vi "MaxX_FITSstacks.vi"() -> ()   [LabVIEW 2011]
panel:
  in  "Skip left":dbl=0.1 min=0.0 max=0.999
  out "error out":errorcluster
  in  "intensity scale factor":dbl=8.0
  out "plane#":i32=24
  out "Intensity Graph":u16[][](graph)
  in  "output folder for 16bit TIFs":path=path "D:/freigabe/MaxX"
  out "fits#":i32=365
  in  "All Files in Dir":path[](array[path])=[path "\\\\BIZ-SERVER\\Messdaten/Entwicklung/Tango/20180703_ISS-flug/AuswertungISS/002_2018-06-21_16-44-14/raw_I000_X0_C0.fits.SIM.fits", path "\\\\BIZ-SERVER\\Messdaten/Entwicklung/Tango/20180703_ISS-flug/AuswertungISS/002_2018-06-21_16-44-14/raw_I000_X0_C1.fits.SIM.fits", path "\\\\BIZ-SERVER\\Messdaten/Entwicklung/Tango/20180703_ISS-flug/AuswertungISS/002_2018-06-21_16-44-14/raw_I000_X0_C3.fits.SIM.fits", path "\\\\BIZ-SERVER\\Messdaten/Entwicklung/Tango/20180703_ISS-flug/AuswertungISS/002_2018-06-21_16-44-14/raw_I000_X1_C0.fits.SIM.fits", path "\\\\BIZ-SERVER\\Messdaten/Entwicklung/Tango/20180703_ISS-flug/AuswertungISS/002_2018-06-21_16-44-14/raw_I000_X1_C3.fits.SIM.fits", path "\\\\BIZ-SERVER\\Messdaten/Entwicklung/Tango/20180703_ISS-flug/AuswertungISS/003_2018-07-03_15-08-29/raw_I000_X0_C0.fits.SIM.fits", path "\\\\BIZ-SERVER\\Messdaten/Entwicklung/Tango/20180703_ISS-flug/AuswertungISS/003_2018-07-03_15-08-29/raw_I000_X0_C1.fits.SIM.fits", path "\\\\BIZ-SERVER\\Messdaten/Entwicklung/Tango/20180703_ISS-flug/AuswertungISS/003_2018-07-03_15-08-29/raw_I000_X0_C3.fits.SIM.fits", path "\\\\BIZ-SERVER\\Messdaten/Entwicklung/Tango/20180703_ISS-flug/AuswertungISS/003_2018-07-03_15-08-29/raw_I000_X1_C0.fits.SIM.fits", path "\\\\BIZ-SERVER\\Messdaten/Entwicklung/Tango/20180703_ISS-flug/AuswertungISS/003_2018-07-03_15-08-29/raw_I000_X1_C3.fits.SIM.fits", path "\\\\BIZ-SERVER\\Messdaten/Entwicklung/Tango/20180703_ISS-flug/AuswertungISS/003_2018-07-03_15-08-29/raw_I001_X1_C0.fits.SIM.fits", path "\\\\BIZ-SERVER\\Messdaten/Entwicklung/Tango/20180703_ISS-flug/AuswertungISS/003_2018-07-03_15-08-29/raw_I001_X1_C3.fits.SIM.fits", path "\\\\BIZ-SERVER\\Messdaten/Entwicklung/Tango/20180703_ISS-flug/AuswertungISS/003_2018-07-03_15-08-29/raw_I002_X1_C0.fits.SIM.fits", path "\\\\BIZ-SERVER\\Messdaten/Entwicklung/Tango/20180703_ISS-flug/AuswertungISS/003_2018-07-03_15-08-29/raw_I002_X1_C3.fits.SIM.fits", path "\\\\BIZ-SERVER\\Messdaten/Entwicklung/Tango/20180703_ISS-flug/AuswertungISS/003_2018-07-03_15-08-29/raw_I003_X1_C0.fits.SIM.fits", path "\\\\BIZ-SERVER\\Messdaten/Entwicklung/Tango/20180703_ISS-flug/AuswertungISS/003_2018-07-03_15-08-29/raw_I003_X1_C3.fits.SIM.fits", path "\\\\BIZ-SERVER\\Messdaten/Entwicklung/Tango/20180703_ISS-flug/AuswertungISS/003_2018-07-03_15-08-29/raw_I004_X1_C0.fits.SIM.fits", path "\\\\BIZ-SERVER\\Messdaten/Entwicklung/Tango/20180703_ISS-flug/AuswertungISS/003_2018-07-03_15-08-29/raw_I004_X1_C3.fits.SIM.fits", path "\\\\BIZ-SERVER\\Messdaten/Entwicklung/Tango/20180703_ISS-flug/AuswertungISS/003_2018-07-03_15-08-29/raw_I005_X1_C0.fits.SIM.fits", path "\\\\BIZ-SERVER\\Messdaten/Entwicklung/Tango/20180703_ISS-flug/AuswertungISS/003_2018-07-03_15-08-29/raw_I005_X1_C3.fits.SIM.fits", path "\\\\BIZ-SERVER\\Messdaten/Entwicklung/Tango/20180703_ISS-flug/AuswertungISS/003_2018-07-03_15-08-29/raw_I006_X1_C0.fits.SIM.fits", path "\\\\BIZ-SERVER\\Messdaten/Entwicklung/Tango/20180703_ISS-flug/AuswertungISS/003_2018-07-03_15-08-29/raw_I006_X1_C3.fits.SIM.fits", path "\\\\BIZ-SERVER\\Messdaten/Entwicklung/Tango/20180703_ISS-flug/AuswertungISS/003_2018-07-03_15-08-29/raw_I007_X1_C0.fits.SIM.fits", path "\\\\BIZ-SERVER\\Messdaten/Entwicklung/Tango/20180703_ISS-flug/AuswertungISS/003_2018-07-03_15-08-29/raw_I007_X1_C3.fits.SIM.fits", path "\\\\BIZ-SERVER\\Messdaten/Entwicklung/Tango/20180703_ISS-flug/AuswertungISS/003_2018-07-03_15-08-29/raw_I008_X1_C0.fits.SIM.fits", path "\\\\BIZ-SERVER\\Messdaten/Entwicklung/Tango/20180703_ISS-flug/AuswertungISS/003_2018-07-03_15-08-29/raw_I008_X1_C3.fits.SIM.fits", path "\\\\BIZ-SERVER\\Messdaten/Entwicklung/Tango/20180703_ISS-flug/AuswertungISS/003_2018-07-03_15-08-29/raw_I009_X0_C0.fits.SIM.fits", path "\\\\BIZ-SERVER\\Messdaten/Entwicklung/Tango/20180703_ISS-flug/AuswertungISS/003_2018-07-03_15-08-29/raw_I009_X0_C1.fits.SIM.fits", path "\\\\BIZ-SERVER\\Messdaten/Entwicklung/Tango/20180703_ISS-flug/AuswertungISS/003_2018-07-03_15-08-29/raw_I009_X0_C3.fits.SIM.fits", path "\\\\BIZ-SERVER\\Messdaten/Entwicklung/Tango/20180703_ISS-flug/AuswertungISS/003_2018-07-03_15-08-29/raw_I009_X1_C0.fits.SIM.fits", path "\\\\BIZ-SERVER\\Messdaten/Entwicklung/Tango/20180703_ISS-flug/AuswertungISS/003_2018-07-03_15-08-29/raw_I009_X1_C3.fits.SIM.fits", path "\\\\BIZ-SERVER\\Messdaten/Entwicklung/Tango/20180703_ISS-flug/AuswertungISS/004_2018-07-03_17-33-15/raw_I000_X0_C0.fits.SIM.fits", path "\\\\BIZ-SERVER\\Messdaten/Entwicklung/Tango/20180703_ISS-flug/AuswertungISS/004_2018-07-03_17-33-15/raw_I000_X0_C1.fits.SIM.fits", path "\\\\BIZ-SERVER\\Messdaten/Entwicklung/Tango/20180703_ISS-flug/AuswertungISS/004_2018-07-03_17-33-15/raw_I000_X0_C3.fits.SIM.fits", path "\\\\BIZ-SERVER\\Messdaten/Entwicklung/Tango/20180703_ISS-flug/AuswertungISS/004_2018-07-03_17-33-15/raw_I000_X1_C0.fits.SIM.fits", path "\\\\BIZ-SERVER\\Messdaten/Entwicklung/Tango/20180703_ISS-flug/AuswertungISS/004_2018-07-03_17-33-15/raw_I000_X1_C3.fits.SIM.fits", path "\\\\BIZ-SERVER\\Messdaten/Entwicklung/Tango/20180703_ISS-flug/AuswertungISS/004_2018-07-03_17-33-15/raw_I001_X1_C0.fits.SIM.fits", path "\\\\BIZ-SERVER\\Messdaten/Entwicklung/Tango/20180703_ISS-flug/AuswertungISS/004_2018-07-03_17-33-15/raw_I001_X1_C3.fits.SIM.fits", path "\\\\BIZ-SERVER\\Messdaten/Entwicklung/Tango/20180703_ISS-flug/AuswertungISS/004_2018-07-03_17-33-15/raw_I002_X1_C0.fits.SIM.fits", path "\\\\BIZ-SERVER\\Messdaten/Entwicklung/Tango/20180703_ISS-flug/AuswertungISS/004_2018-07-03_17-33-15/raw_I002_X1_C3.fits.SIM.fits", path "\\\\BIZ-SERVER\\Messdaten/Entwicklung/Tango/20180703_ISS-flug/AuswertungISS/004_2018-07-03_17-33-15/raw_I003_X1_C0.fits.SIM.fits", path "\\\\BIZ-SERVER\\Messdaten/Entwicklung/Tango/20180703_ISS-flug/AuswertungISS/004_2018-07-03_17-33-15/raw_I003_X1_C3.fits.SIM.fits", path "\\\\BIZ-SERVER\\Messdaten/Entwicklung/Tango/20180703_ISS-flug/AuswertungISS/004_2018-07-03_17-33-15/raw_I004_X1_C0.fits.SIM.fits", path "\\\\BIZ-SERVER\\Messdaten/Entwicklung/Tango/20180703_ISS-flug/AuswertungISS/004_2018-07-03_17-33-15/raw_I004_X1_C3.fits.SIM.fits", path "\\\\BIZ-SERVER\\Messdaten/Entwicklung/Tango/20180703_ISS-flug/AuswertungISS/004_2018-07-03_17-33-15/raw_I005_X1_C0.fits.SIM.fits", path "\\\\BIZ-SERVER\\Messdaten/Entwicklung/Tango/20180703_ISS-flug/AuswertungISS/004_2018-07-03_17-33-15/raw_I005_X1_C3.fits.SIM.fits", path "\\\\BIZ-SERVER\\Messdaten/Entwicklung/Tango/20180703_ISS-flug/AuswertungISS/004_2018-07-03_17-33-15/raw_I006_X1_C0.fits.SIM.fits", path "\\\\BIZ-SERVER\\Messdaten/Entwicklung/Tango/20180703_ISS-flug/AuswertungISS/004_2018-07-03_17-33-15/raw_I006_X1_C3.fits.SIM.fits", path "\\\\BIZ-SERVER\\Messdaten/Entwicklung/Tango/20180703_ISS-flug/AuswertungISS/004_2018-07-03_17-33-15/raw_I007_X1_C0.fits.SIM.fits", path "\\\\BIZ-SERVER\\Messdaten/Entwicklung/Tango/20180703_ISS-flug/AuswertungISS/004_2018-07-03_17-33-15/raw_I007_X1_C3.fits.SIM.fits", path "\\\\BIZ-SERVER\\Messdaten/Entwicklung/Tango/20180703_ISS-flug/AuswertungISS/004_2018-07-03_17-33-15/raw_I008_X1_C0.fits.SIM.fits", path "\\\\BIZ-SERVER\\Messdaten/Entwicklung/Tango/20180703_ISS-flug/AuswertungISS/004_2018-07-03_17-33-15/raw_I008_X1_C3.fits.SIM.fits", path "\\\\BIZ-SERVER\\Messdaten/Entwicklung/Tango/20180703_ISS-flug/AuswertungISS/004_2018-07-03_17-33-15/raw_I009_X1_C0.fits.SIM.fits", path "\\\\BIZ-SERVER\\Messdaten/Entwicklung/Tango/20180703_ISS-flug/AuswertungISS/004_2018-07-03_17-33-15/raw_I009_X1_C3.fits.SIM.fits", path "\\\\BIZ-SERVER\\Messdaten/Entwicklung/Tango/20180703_ISS-flug/AuswertungISS/004_2018-07-03_17-33-15/raw_I010_X1_C0.fits.SIM.fits", path "\\\\BIZ-SERVER\\Messdaten/Entwicklung/Tango/20180703_ISS-flug/AuswertungISS/004_2018-07-03_17-33-15/raw_I010_X1_C3.fits.SIM.fits", path "\\\\BIZ-SERVER\\Messdaten/Entwicklung/Tango/20180703_ISS-flug/AuswertungISS/004_2018-07-03_17-33-15/raw_I011_X1_C0.fits.SIM.fits", path "\\\\BIZ-SERVER\\Messdaten/Entwicklung/Tango/20180703_ISS-flug/AuswertungISS/004_2018-07-03_17-33-15/raw_I011_X1_C3.fits.SIM.fits", path "\\\\BIZ-SERVER\\Messdaten/Entwicklung/Tango/20180703_ISS-flug/AuswertungISS/004_2018-07-03_17-33-15/raw_I012_X1_C0.fits.SIM.fits", path "\\\\BIZ-SERVER\\Messdaten/Entwicklung/Tango/20180703_ISS-flug/AuswertungISS/004_2018-07-03_17-33-15/raw_I012_X1_C3.fits.SIM.fits", path "\\\\BIZ-SERVER\\Messdaten/Entwicklung/Tango/20180703_ISS-flug/AuswertungISS/004_2018-07-03_17-33-15/raw_I013_X1_C0.fits.SIM.fits", path "\\\\BIZ-SERVER\\Messdaten/Entwicklung/Tango/20180703_ISS-flug/AuswertungISS/004_2018-07-03_17-33-15/raw_I013_X1_C3.fits.SIM.fits", path "\\\\BIZ-SERVER\\Messdaten/Entwicklung/Tango/20180703_ISS-flug/AuswertungISS/004_2018-07-03_17-33-15/raw_I014_X1_C0.fits.SIM.fits", path "\\\\BIZ-SERVER\\Messdaten/Entwicklung/Tango/20180703_ISS-flug/AuswertungISS/004_2018-07-03_17-33-15/raw_I014_X1_C3.fits.SIM.fits", path "\\\\BIZ-SERVER\\Messdaten/Entwicklung/Tango/20180703_ISS-flug/AuswertungISS/004_2018-07-03_17-33-15/raw_I015_X1_C0.fits.SIM.fits", path "\\\\BIZ-SERVER\\Messdaten/Entwicklung/Tango/20180703_ISS-flug/AuswertungISS/004_2018-07-03_17-33-15/raw_I015_X1_C3.fits.SIM.fits", path "\\\\BIZ-SERVER\\Messdaten/Entwicklung/Tango/20180703_ISS-flug/AuswertungISS/004_2018-07-03_17-33-15/raw_I016_X1_C0.fits.SIM.fits", path "\\\\BIZ-SERVER\\Messdaten/Entwicklung/Tango/20180703_ISS-flug/AuswertungISS/004_2018-07-03_17-33-15/raw_I016_X1_C3.fits.SIM.fits", path "\\\\BIZ-SERVER\\Messdaten/Entwicklung/Tango/20180703_ISS-flug/AuswertungISS/004_2018-07-03_17-33-15/raw_I017_X1_C0.fits.SIM.fits", path "\\\\BIZ-SERVER\\Messdaten/Entwicklung/Tango/20180703_ISS-flug/AuswertungISS/004_2018-07-03_17-33-15/raw_I017_X1_C3.fits.SIM.fits", path "\\\\BIZ-SERVER\\Messdaten/Entwicklung/Tango/20180703_ISS-flug/AuswertungISS/005_2018-07-04_08-02-54/raw_I000_X0_C0.fits.SIM.fits", path "\\\\BIZ-SERVER\\Messdaten/Entwicklung/Tango/20180703_ISS-flug/AuswertungISS/005_2018-07-04_08-02-54/raw_I000_X0_C1.fits.SIM.fits", path "\\\\BIZ-SERVER\\Messdaten/Entwicklung/Tango/20180703_ISS-flug/AuswertungISS/005_2018-07-04_08-02-54/raw_I000_X0_C3.fits.SIM.fits", path "\\\\BIZ-SERVER\\Messdaten/Entwicklung/Tango/20180703_ISS-flug/AuswertungISS/005_2018-07-04_08-02-54/raw_I000_X1_C0.fits.SIM.fits", path "\\\\BIZ-SERVER\\Messdaten/Entwicklung/Tango/20180703_ISS-flug/AuswertungISS/005_2018-07-04_08-02-54/raw_I000_X1_C3.fits.SIM.fits", path "\\\\BIZ-SERVER\\Messdaten/Entwicklung/Tango/20180703_ISS-flug/AuswertungISS/005_2018-07-04_08-02-54/raw_I001_X1_C0.fits.SIM.fits", path "\\\\BIZ-SERVER\\Messdaten/Entwicklung/Tango/20180703_ISS-flug/AuswertungISS/005_2018-07-04_08-02-54/raw_I001_X1_C3.fits.SIM.fits", path "\\\\BIZ-SERVER\\Messdaten/Entwicklung/Tango/20180703_ISS-flug/AuswertungISS/005_2018-07-04_08-02-54/raw_I002_X1_C0.fits.SIM.fits", path "\\\\BIZ-SERVER\\Messdaten/Entwicklung/Tango/20180703_ISS-flug/AuswertungISS/005_2018-07-04_08-02-54/raw_I002_X1_C3.fits.SIM.fits", path "\\\\BIZ-SERVER\\Messdaten/Entwicklung/Tango/20180703_ISS-flug/AuswertungISS/005_2018-07-04_08-02-54/raw_I003_X1_C0.fits.SIM.fits", path "\\\\BIZ-SERVER\\Messdaten/Entwicklung/Tango/20180703_ISS-flug/AuswertungISS/005_2018-07-04_08-02-54/raw_I003_X1_C3.fits.SIM.fits", path "\\\\BIZ-SERVER\\Messdaten/Entwicklung/Tango/20180703_ISS-flug/AuswertungISS/005_2018-07-04_08-02-54/raw_I004_X1_C0.fits.SIM.fits", path "\\\\BIZ-SERVER\\Messdaten/Entwicklung/Tango/20180703_ISS-flug/AuswertungISS/005_2018-07-04_08-02-54/raw_I004_X1_C3.fits.SIM.fits", path "\\\\BIZ-SERVER\\Messdaten/Entwicklung/Tango/20180703_ISS-flug/AuswertungISS/005_2018-07-04_08-02-54/raw_I005_X1_C0.fits.SIM.fits", path "\\\\BIZ-SERVER\\Messdaten/Entwicklung/Tango/20180703_ISS-flug/AuswertungISS/005_2018-07-04_08-02-54/raw_I005_X1_C3.fits.SIM.fits", path "\\\\BIZ-SERVER\\Messdaten/Entwicklung/Tango/20180703_ISS-flug/AuswertungISS/005_2018-07-04_08-02-54/raw_I006_X1_C0.fits.SIM.fits", path "\\\\BIZ-SERVER\\Messdaten/Entwicklung/Tango/20180703_ISS-flug/AuswertungISS/005_2018-07-04_08-02-54/raw_I006_X1_C3.fits.SIM.fits", path "\\\\BIZ-SERVER\\Messdaten/Entwicklung/Tango/20180703_ISS-flug/AuswertungISS/005_2018-07-04_08-02-54/raw_I007_X1_C0.fits.SIM.fits", path "\\\\BIZ-SERVER\\Messdaten/Entwicklung/Tango/20180703_ISS-flug/AuswertungISS/005_2018-07-04_08-02-54/raw_I007_X1_C3.fits.SIM.fits", path "\\\\BIZ-SERVER\\Messdaten/Entwicklung/Tango/20180703_ISS-flug/AuswertungISS/005_2018-07-04_08-02-54/raw_I008_X1_C0.fits.SIM.fits", path "\\\\BIZ-SERVER\\Messdaten/Entwicklung/Tango/20180703_ISS-flug/AuswertungISS/005_2018-07-04_08-02-54/raw_I008_X1_C3.fits.SIM.fits", path "\\\\BIZ-SERVER\\Messdaten/Entwicklung/Tango/20180703_ISS-flug/AuswertungISS/005_2018-07-04_08-02-54/raw_I009_X1_C0.fits.SIM.fits", path "\\\\BIZ-SERVER\\Messdaten/Entwicklung/Tango/20180703_ISS-flug/AuswertungISS/005_2018-07-04_08-02-54/raw_I009_X1_C3.fits.SIM.fits", path "\\\\BIZ-SERVER\\Messdaten/Entwicklung/Tango/20180703_ISS-flug/AuswertungISS/005_2018-07-04_08-02-54/raw_I010_X1_C0.fits.SIM.fits", path "\\\\BIZ-SERVER\\Messdaten/Entwicklung/Tango/20180703_ISS-flug/AuswertungISS/005_2018-07-04_08-02-54/raw_I010_X1_C3.fits.SIM.fits", path "\\\\BIZ-SERVER\\Messdaten/Entwicklung/Tango/20180703_ISS-flug/AuswertungISS/005_2018-07-04_08-02-54/raw_I011_X1_C0.fits.SIM.fits", path "\\\\BIZ-SERVER\\Messdaten/Entwicklung/Tango/20180703_ISS-flug/AuswertungISS/005_2018-07-04_08-02-54/raw_I011_X1_C3.fits.SIM.fits", path "\\\\BIZ-SERVER\\Messdaten/Entwicklung/Tango/20180703_ISS-flug/AuswertungISS/005_2018-07-04_08-02-54/raw_I012_X1_C0.fits.SIM.fits", path "\\\\BIZ-SERVER\\Messdaten/Entwicklung/Tango/20180703_ISS-flug/AuswertungISS/005_2018-07-04_08-02-54/raw_I012_X1_C3.fits.SIM.fits", path "\\\\BIZ-SERVER\\Messdaten/Entwicklung/Tango/20180703_ISS-flug/AuswertungISS/005_2018-07-04_08-02-54/raw_I013_X1_C0.fits.SIM.fits", path "\\\\BIZ-SERVER\\Messdaten/Entwicklung/Tango/20180703_ISS-flug/AuswertungISS/005_2018-07-04_08-02-54/raw_I013_X1_C3.fits.SIM.fits", path "\\\\BIZ-SERVER\\Messdaten/Entwicklung/Tango/20180703_ISS-flug/AuswertungISS/005_2018-07-04_08-02-54/raw_I014_X1_C0.fits.SIM.fits", path "\\\\BIZ-SERVER\\Messdaten/Entwicklung/Tango/20180703_ISS-flug/AuswertungISS/005_2018-07-04_08-02-54/raw_I014_X1_C3.fits.SIM.fits", path "\\\\BIZ-SERVER\\Messdaten/Entwicklung/Tango/20180703_ISS-flug/AuswertungISS/005_2018-07-04_08-02-54/raw_I015_X1_C0.fits.SIM.fits", path "\\\\BIZ-SERVER\\Messdaten/Entwicklung/Tango/20180703_ISS-flug/AuswertungISS/005_2018-07-04_08-02-54/raw_I015_X1_C3.fits.SIM.fits", path "\\\\BIZ-SERVER\\Messdaten/Entwicklung/Tango/20180703_ISS-flug/AuswertungISS/005_2018-07-04_08-02-54/raw_I016_X1_C0.fits.SIM.fits", path "\\\\BIZ-SERVER\\Messdaten/Entwicklung/Tango/20180703_ISS-flug/AuswertungISS/005_2018-07-04_08-02-54/raw_I016_X1_C3.fits.SIM.fits", path "\\\\BIZ-SERVER\\Messdaten/Entwicklung/Tango/20180703_ISS-flug/AuswertungISS/006_2018-07-04_15-43-18/raw_I000_X0_C0.fits.SIM.fits", path "\\\\BIZ-SERVER\\Messdaten/Entwicklung/Tango/20180703_ISS-flug/AuswertungISS/006_2018-07-04_15-43-18/raw_I000_X0_C1.fits.SIM.fits", path "\\\\BIZ-SERVER\\Messdaten/Entwicklung/Tango/20180703_ISS-flug/AuswertungISS/006_2018-07-04_15-43-18/raw_I000_X0_C3.fits.SIM.fits", path "\\\\BIZ-SERVER\\Messdaten/Entwicklung/Tango/20180703_ISS-flug/AuswertungISS/006_2018-07-04_15-43-18/raw_I000_X1_C0.fits.SIM.fits", path "\\\\BIZ-SERVER\\Messdaten/Entwicklung/Tango/20180703_ISS-flug/AuswertungISS/006_2018-07-04_15-43-18/raw_I000_X1_C3.fits.SIM.fits", path "\\\\BIZ-SERVER\\Messdaten/Entwicklung/Tango/20180703_ISS-flug/AuswertungISS/006_2018-07-04_15-43-18/raw_I001_X1_C0.fits.SIM.fits", path "\\\\BIZ-SERVER\\Messdaten/Entwicklung/Tango/20180703_ISS-flug/AuswertungISS/006_2018-07-04_15-43-18/raw_I001_X1_C3.fits.SIM.fits", path "\\\\BIZ-SERVER\\Messdaten/Entwicklung/Tango/20180703_ISS-flug/AuswertungISS/006_2018-07-04_15-43-18/raw_I002_X1_C0.fits.SIM.fits", path "\\\\BIZ-SERVER\\Messdaten/Entwicklung/Tango/20180703_ISS-flug/AuswertungISS/006_2018-07-04_15-43-18/raw_I002_X1_C3.fits.SIM.fits", path "\\\\BIZ-SERVER\\Messdaten/Entwicklung/Tango/20180703_ISS-flug/AuswertungISS/006_2018-07-04_15-43-18/raw_I003_X1_C0.fits.SIM.fits", path "\\\\BIZ-SERVER\\Messdaten/Entwicklung/Tango/20180703_ISS-flug/AuswertungISS/006_2018-07-04_15-43-18/raw_I003_X1_C3.fits.SIM.fits", path "\\\\BIZ-SERVER\\Messdaten/Entwicklung/Tango/20180703_ISS-flug/AuswertungISS/007_2018-07-04_16-44-22/raw_I000_X0_C0.fits.SIM.fits", path "\\\\BIZ-SERVER\\Messdaten/Entwicklung/Tango/20180703_ISS-flug/AuswertungISS/007_2018-07-04_16-44-22/raw_I000_X0_C1.fits.SIM.fits", path "\\\\BIZ-SERVER\\Messdaten/Entwicklung/Tango/20180703_ISS-flug/AuswertungISS/007_2018-07-04_16-44-22/raw_I000_X0_C3.fits.SIM.fits", path "\\\\BIZ-SERVER\\Messdaten/Entwicklung/Tango/20180703_ISS-flug/AuswertungISS/007_2018-07-04_16-44-22/raw_I000_X1_C0.fits.SIM.fits", path "\\\\BIZ-SERVER\\Messdaten/Entwicklung/Tango/20180703_ISS-flug/AuswertungISS/007_2018-07-04_16-44-22/raw_I000_X1_C3.fits.SIM.fits", path "\\\\BIZ-SERVER\\Messdaten/Entwicklung/Tango/20180703_ISS-flug/AuswertungISS/007_2018-07-04_16-44-22/raw_I001_X1_C0.fits.SIM.fits", path "\\\\BIZ-SERVER\\Messdaten/Entwicklung/Tango/20180703_ISS-flug/AuswertungISS/007_2018-07-04_16-44-22/raw_I001_X1_C3.fits.SIM.fits", path "\\\\BIZ-SERVER\\Messdaten/Entwicklung/Tango/20180703_ISS-flug/AuswertungISS/007_2018-07-04_16-44-22/raw_I002_X1_C0.fits.SIM.fits", path "\\\\BIZ-SERVER\\Messdaten/Entwicklung/Tango/20180703_ISS-flug/AuswertungISS/007_2018-07-04_16-44-22/raw_I002_X1_C3.fits.SIM.fits", path "\\\\BIZ-SERVER\\Messdaten/Entwicklung/Tango/20180703_ISS-flug/AuswertungISS/007_2018-07-04_16-44-22/raw_I003_X1_C0.fits.SIM.fits", path "\\\\BIZ-SERVER\\Messdaten/Entwicklung/Tango/20180703_ISS-flug/AuswertungISS/007_2018-07-04_16-44-22/raw_I003_X1_C3.fits.SIM.fits", path "\\\\BIZ-SERVER\\Messdaten/Entwicklung/Tango/20180703_ISS-flug/AuswertungISS/007_2018-07-04_16-44-22/raw_I004_X1_C0.fits.SIM.fits", path "\\\\BIZ-SERVER\\Messdaten/Entwicklung/Tango/20180703_ISS-flug/AuswertungISS/007_2018-07-04_16-44-22/raw_I004_X1_C3.fits.SIM.fits", path "\\\\BIZ-SERVER\\Messdaten/Entwicklung/Tango/20180703_ISS-flug/AuswertungISS/007_2018-07-04_16-44-22/raw_I005_X1_C0.fits.SIM.fits", path "\\\\BIZ-SERVER\\Messdaten/Entwicklung/Tango/20180703_ISS-flug/AuswertungISS/007_2018-07-04_16-44-22/raw_I005_X1_C3.fits.SIM.fits", path "\\\\BIZ-SERVER\\Messdaten/Entwicklung/Tango/20180703_ISS-flug/AuswertungISS/007_2018-07-04_16-44-22/raw_I006_X1_C0.fits.SIM.fits", path "\\\\BIZ-SERVER\\Messdaten/Entwicklung/Tango/20180703_ISS-flug/AuswertungISS/007_2018-07-04_16-44-22/raw_I006_X1_C3.fits.SIM.fits", path "\\\\BIZ-SERVER\\Messdaten/Entwicklung/Tango/20180703_ISS-flug/AuswertungISS/007_2018-07-04_16-44-22/raw_I007_X1_C0.fits.SIM.fits", path "\\\\BIZ-SERVER\\Messdaten/Entwicklung/Tango/20180703_ISS-flug/AuswertungISS/007_2018-07-04_16-44-22/raw_I007_X1_C3.fits.SIM.fits", path "\\\\BIZ-SERVER\\Messdaten/Entwicklung/Tango/20180703_ISS-flug/AuswertungISS/007_2018-07-04_16-44-22/raw_I008_X1_C0.fits.SIM.fits", path "\\\\BIZ-SERVER\\Messdaten/Entwicklung/Tango/20180703_ISS-flug/AuswertungISS/007_2018-07-04_16-44-22/raw_I008_X1_C3.fits.SIM.fits", path "\\\\BIZ-SERVER\\Messdaten/Entwicklung/Tango/20180703_ISS-flug/AuswertungISS/007_2018-07-04_16-44-22/raw_I009_X1_C0.fits.SIM.fits", path "\\\\BIZ-SERVER\\Messdaten/Entwicklung/Tango/20180703_ISS-flug/AuswertungISS/007_2018-07-04_16-44-22/raw_I009_X1_C3.fits.SIM.fits", path "\\\\BIZ-SERVER\\Messdaten/Entwicklung/Tango/20180703_ISS-flug/AuswertungISS/007_2018-07-04_16-44-22/raw_I010_X1_C0.fits.SIM.fits", path "\\\\BIZ-SERVER\\Messdaten/Entwicklung/Tango/20180703_ISS-flug/AuswertungISS/007_2018-07-04_16-44-22/raw_I010_X1_C3.fits.SIM.fits", path "\\\\BIZ-SERVER\\Messdaten/Entwicklung/Tango/20180703_ISS-flug/AuswertungISS/007_2018-07-04_16-44-22/raw_I011_X1_C0.fits.SIM.fits", path "\\\\BIZ-SERVER\\Messdaten/Entwicklung/Tango/20180703_ISS-flug/AuswertungISS/007_2018-07-04_16-44-22/raw_I011_X1_C3.fits.SIM.fits", path "\\\\BIZ-SERVER\\Messdaten/Entwicklung/Tango/20180703_ISS-flug/AuswertungISS/007_2018-07-04_16-44-22/raw_I012_X1_C0.fits.SIM.fits", path "\\\\BIZ-SERVER\\Messdaten/Entwicklung/Tango/20180703_ISS-flug/AuswertungISS/007_2018-07-04_16-44-22/raw_I012_X1_C3.fits.SIM.fits", path "\\\\BIZ-SERVER\\Messdaten/Entwicklung/Tango/20180703_ISS-flug/AuswertungISS/007_2018-07-04_16-44-22/raw_I013_X1_C0.fits.SIM.fits", path "\\\\BIZ-SERVER\\Messdaten/Entwicklung/Tango/20180703_ISS-flug/AuswertungISS/007_2018-07-04_16-44-22/raw_I013_X1_C3.fits.SIM.fits", path "\\\\BIZ-SERVER\\Messdaten/Entwicklung/Tango/20180703_ISS-flug/AuswertungISS/007_2018-07-04_16-44-22/raw_I014_X1_C0.fits.SIM.fits", path "\\\\BIZ-SERVER\\Messdaten/Entwicklung/Tango/20180703_ISS-flug/AuswertungISS/007_2018-07-04_16-44-22/raw_I014_X1_C3.fits.SIM.fits", path "\\\\BIZ-SERVER\\Messdaten/Entwicklung/Tango/20180703_ISS-flug/AuswertungISS/007_2018-07-04_16-44-22/raw_I015_X1_C0.fits.SIM.fits", path "\\\\BIZ-SERVER\\Messdaten/Entwicklung/Tango/20180703_ISS-flug/AuswertungISS/007_2018-07-04_16-44-22/raw_I015_X1_C3.fits.SIM.fits", path "\\\\BIZ-SERVER\\Messdaten/Entwicklung/Tango/20180703_ISS-flug/AuswertungISS/007_2018-07-04_16-44-22/raw_I016_X1_C0.fits.SIM.fits", path "\\\\BIZ-SERVER\\Messdaten/Entwicklung/Tango/20180703_ISS-flug/AuswertungISS/007_2018-07-04_16-44-22/raw_I016_X1_C3.fits.SIM.fits", path "\\\\BIZ-SERVER\\Messdaten/Entwicklung/Tango/20180703_ISS-flug/AuswertungISS/007_2018-07-04_16-44-22/raw_I017_X1_C0.fits.SIM.fits", path "\\\\BIZ-SERVER\\Messdaten/Entwicklung/Tango/20180703_ISS-flug/AuswertungISS/007_2018-07-04_16-44-22/raw_I017_X1_C3.fits.SIM.fits", path "\\\\BIZ-SERVER\\Messdaten/Entwicklung/Tango/20180703_ISS-flug/AuswertungISS/008_2018-07-05_08-02-52/raw_I000_X0_C0.fits.SIM.fits", path "\\\\BIZ-SERVER\\Messdaten/Entwicklung/Tango/20180703_ISS-flug/AuswertungISS/008_2018-07-05_08-02-52/raw_I000_X0_C1.fits.SIM.fits", path "\\\\BIZ-SERVER\\Messdaten/Entwicklung/Tango/20180703_ISS-flug/AuswertungISS/008_2018-07-05_08-02-52/raw_I000_X0_C3.fits.SIM.fits", path "\\\\BIZ-SERVER\\Messdaten/Entwicklung/Tango/20180703_ISS-flug/AuswertungISS/008_2018-07-05_08-02-52/raw_I000_X1_C0.fits.SIM.fits", path "\\\\BIZ-SERVER\\Messdaten/Entwicklung/Tango/20180703_ISS-flug/AuswertungISS/008_2018-07-05_08-02-52/raw_I000_X1_C3.fits.SIM.fits", path "\\\\BIZ-SERVER\\Messdaten/Entwicklung/Tango/20180703_ISS-flug/AuswertungISS/008_2018-07-05_08-02-52/raw_I001_X1_C0.fits.SIM.fits", path "\\\\BIZ-SERVER\\Messdaten/Entwicklung/Tango/20180703_ISS-flug/AuswertungISS/008_2018-07-05_08-02-52/raw_I001_X1_C3.fits.SIM.fits", path "\\\\BIZ-SERVER\\Messdaten/Entwicklung/Tango/20180703_ISS-flug/AuswertungISS/008_2018-07-05_08-02-52/raw_I002_X1_C0.fits.SIM.fits", path "\\\\BIZ-SERVER\\Messdaten/Entwicklung/Tango/20180703_ISS-flug/AuswertungISS/008_2018-07-05_08-02-52/raw_I002_X1_C3.fits.SIM.fits", path "\\\\BIZ-SERVER\\Messdaten/Entwicklung/Tango/20180703_ISS-flug/AuswertungISS/008_2018-07-05_08-02-52/raw_I003_X1_C0.fits.SIM.fits", path "\\\\BIZ-SERVER\\Messdaten/Entwicklung/Tango/20180703_ISS-flug/AuswertungISS/008_2018-07-05_08-02-52/raw_I003_X1_C3.fits.SIM.fits", path "\\\\BIZ-SERVER\\Messdaten/Entwicklung/Tango/20180703_ISS-flug/AuswertungISS/008_2018-07-05_08-02-52/raw_I004_X1_C0.fits.SIM.fits", path "\\\\BIZ-SERVER\\Messdaten/Entwicklung/Tango/20180703_ISS-flug/AuswertungISS/008_2018-07-05_08-02-52/raw_I004_X1_C3.fits.SIM.fits", path "\\\\BIZ-SERVER\\Messdaten/Entwicklung/Tango/20180703_ISS-flug/AuswertungISS/008_2018-07-05_08-02-52/raw_I005_X1_C0.fits.SIM.fits", path "\\\\BIZ-SERVER\\Messdaten/Entwicklung/Tango/20180703_ISS-flug/AuswertungISS/008_2018-07-05_08-02-52/raw_I005_X1_C3.fits.SIM.fits", path "\\\\BIZ-SERVER\\Messdaten/Entwicklung/Tango/20180703_ISS-flug/AuswertungISS/008_2018-07-05_08-02-52/raw_I006_X1_C0.fits.SIM.fits", path "\\\\BIZ-SERVER\\Messdaten/Entwicklung/Tango/20180703_ISS-flug/AuswertungISS/008_2018-07-05_08-02-52/raw_I006_X1_C3.fits.SIM.fits", path "\\\\BIZ-SERVER\\Messdaten/Entwicklung/Tango/20180703_ISS-flug/AuswertungISS/008_2018-07-05_08-02-52/raw_I007_X1_C0.fits.SIM.fits", path "\\\\BIZ-SERVER\\Messdaten/Entwicklung/Tango/20180703_ISS-flug/AuswertungISS/008_2018-07-05_08-02-52/raw_I007_X1_C3.fits.SIM.fits", path "\\\\BIZ-SERVER\\Messdaten/Entwicklung/Tango/20180703_ISS-flug/AuswertungISS/008_2018-07-05_08-02-52/raw_I008_X1_C0.fits.SIM.fits", path "\\\\BIZ-SERVER\\Messdaten/Entwicklung/Tango/20180703_ISS-flug/AuswertungISS/008_2018-07-05_08-02-52/raw_I008_X1_C3.fits.SIM.fits", path "\\\\BIZ-SERVER\\Messdaten/Entwicklung/Tango/20180703_ISS-flug/AuswertungISS/008_2018-07-05_08-02-52/raw_I009_X1_C0.fits.SIM.fits", path "\\\\BIZ-SERVER\\Messdaten/Entwicklung/Tango/20180703_ISS-flug/AuswertungISS/008_2018-07-05_08-02-52/raw_I009_X1_C3.fits.SIM.fits", path "\\\\BIZ-SERVER\\Messdaten/Entwicklung/Tango/20180703_ISS-flug/AuswertungISS/008_2018-07-05_08-02-52/raw_I010_X1_C0.fits.SIM.fits", path "\\\\BIZ-SERVER\\Messdaten/Entwicklung/Tango/20180703_ISS-flug/AuswertungISS/008_2018-07-05_08-02-52/raw_I010_X1_C3.fits.SIM.fits", path "\\\\BIZ-SERVER\\Messdaten/Entwicklung/Tango/20180703_ISS-flug/AuswertungISS/008_2018-07-05_08-02-52/raw_I011_X1_C0.fits.SIM.fits", path "\\\\BIZ-SERVER\\Messdaten/Entwicklung/Tango/20180703_ISS-flug/AuswertungISS/008_2018-07-05_08-02-52/raw_I011_X1_C3.fits.SIM.fits", path "\\\\BIZ-SERVER\\Messdaten/Entwicklung/Tango/20180703_ISS-flug/AuswertungISS/008_2018-07-05_08-02-52/raw_I012_X1_C0.fits.SIM.fits", path "\\\\BIZ-SERVER\\Messdaten/Entwicklung/Tango/20180703_ISS-flug/AuswertungISS/008_2018-07-05_08-02-52/raw_I012_X1_C3.fits.SIM.fits", path "\\\\BIZ-SERVER\\Messdaten/Entwicklung/Tango/20180703_ISS-flug/AuswertungISS/008_2018-07-05_08-02-52/raw_I013_X1_C0.fits.SIM.fits", path "\\\\BIZ-SERVER\\Messdaten/Entwicklung/Tango/20180703_ISS-flug/AuswertungISS/008_2018-07-05_08-02-52/raw_I013_X1_C3.fits.SIM.fits", path "\\\\BIZ-SERVER\\Messdaten/Entwicklung/Tango/20180703_ISS-flug/AuswertungISS/008_2018-07-05_08-02-52/raw_I014_X1_C0.fits.SIM.fits", path "\\\\BIZ-SERVER\\Messdaten/Entwicklung/Tango/20180703_ISS-flug/AuswertungISS/008_2018-07-05_08-02-52/raw_I014_X1_C3.fits.SIM.fits", path "\\\\BIZ-SERVER\\Messdaten/Entwicklung/Tango/20180703_ISS-flug/AuswertungISS/008_2018-07-05_08-02-52/raw_I015_X1_C0.fits.SIM.fits", path "\\\\BIZ-SERVER\\Messdaten/Entwicklung/Tango/20180703_ISS-flug/AuswertungISS/008_2018-07-05_08-02-52/raw_I015_X1_C3.fits.SIM.fits", path "\\\\BIZ-SERVER\\Messdaten/Entwicklung/Tango/20180703_ISS-flug/AuswertungISS/008_2018-07-05_08-02-52/raw_I016_X1_C0.fits.SIM.fits", path "\\\\BIZ-SERVER\\Messdaten/Entwicklung/Tango/20180703_ISS-flug/AuswertungISS/008_2018-07-05_08-02-52/raw_I016_X1_C3.fits.SIM.fits", path "\\\\BIZ-SERVER\\Messdaten/Entwicklung/Tango/20180703_ISS-flug/AuswertungISS/008_2018-07-05_08-02-52/raw_I017_X1_C0.fits.SIM.fits", path "\\\\BIZ-SERVER\\Messdaten/Entwicklung/Tango/20180703_ISS-flug/AuswertungISS/008_2018-07-05_08-02-52/raw_I017_X1_C3.fits.SIM.fits", path "\\\\BIZ-SERVER\\Messdaten/Entwicklung/Tango/20180703_ISS-flug/AuswertungISS/009_2018-07-05_20-57-36/raw_I000_X0_C0.fits.SIM.fits", path "\\\\BIZ-SERVER\\Messdaten/Entwicklung/Tango/20180703_ISS-flug/AuswertungISS/009_2018-07-05_20-57-36/raw_I000_X0_C1.fits.SIM.fits", path "\\\\BIZ-SERVER\\Messdaten/Entwicklung/Tango/20180703_ISS-flug/AuswertungISS/009_2018-07-05_20-57-36/raw_I000_X0_C3.fits.SIM.fits", path "\\\\BIZ-SERVER\\Messdaten/Entwicklung/Tango/20180703_ISS-flug/AuswertungISS/009_2018-07-05_20-57-36/raw_I000_X1_C3.fits.SIM.fits", path "\\\\BIZ-SERVER\\Messdaten/Entwicklung/Tango/20180703_ISS-flug/AuswertungISS/009_2018-07-05_20-57-36/raw_I001_X1_C3.fits.SIM.fits", path "\\\\BIZ-SERVER\\Messdaten/Entwicklung/Tango/20180703_ISS-flug/AuswertungISS/009_2018-07-05_20-57-36/raw_I002_X1_C3.fits.SIM.fits", path "\\\\BIZ-SERVER\\Messdaten/Entwicklung/Tango/20180703_ISS-flug/AuswertungISS/009_2018-07-05_20-57-36/raw_I003_X1_C3.fits.SIM.fits", path "\\\\BIZ-SERVER\\Messdaten/Entwicklung/Tango/20180703_ISS-flug/AuswertungISS/009_2018-07-05_20-57-36/raw_I004_X1_C3.fits.SIM.fits", path "\\\\BIZ-SERVER\\Messdaten/Entwicklung/Tango/20180703_ISS-flug/AuswertungISS/009_2018-07-05_20-57-36/raw_I005_X1_C3.fits.SIM.fits", path "\\\\BIZ-SERVER\\Messdaten/Entwicklung/Tango/20180703_ISS-flug/AuswertungISS/009_2018-07-05_20-57-36/raw_I006_X1_C3.fits.SIM.fits", path "\\\\BIZ-SERVER\\Messdaten/Entwicklung/Tango/20180703_ISS-flug/AuswertungISS/009_2018-07-05_20-57-36/raw_I007_X1_C3.fits.SIM.fits", path "\\\\BIZ-SERVER\\Messdaten/Entwicklung/Tango/20180703_ISS-flug/AuswertungISS/009_2018-07-05_20-57-36/raw_I008_X1_C3.fits.SIM.fits", path "\\\\BIZ-SERVER\\Messdaten/Entwicklung/Tango/20180703_ISS-flug/AuswertungISS/009_2018-07-05_20-57-36/raw_I009_X1_C3.fits.SIM.fits", path "\\\\BIZ-SERVER\\Messdaten/Entwicklung/Tango/20180703_ISS-flug/AuswertungISS/009_2018-07-05_20-57-36/raw_I010_X1_C3.fits.SIM.fits", path "\\\\BIZ-SERVER\\Messdaten/Entwicklung/Tango/20180703_ISS-flug/AuswertungISS/009_2018-07-05_20-57-36/raw_I011_X1_C3.fits.SIM.fits", path "\\\\BIZ-SERVER\\Messdaten/Entwicklung/Tango/20180703_ISS-flug/AuswertungISS/010_2018-07-06_17-20-26/raw_I000_X0_C0.fits.SIM.fits", path "\\\\BIZ-SERVER\\Messdaten/Entwicklung/Tango/20180703_ISS-flug/AuswertungISS/010_2018-07-06_17-20-26/raw_I000_X0_C1.fits.SIM.fits", path "\\\\BIZ-SERVER\\Messdaten/Entwicklung/Tango/20180703_ISS-flug/AuswertungISS/010_2018-07-06_17-20-26/raw_I000_X0_C3.fits.SIM.fits", path "\\\\BIZ-SERVER\\Messdaten/Entwicklung/Tango/20180703_ISS-flug/AuswertungISS/010_2018-07-06_17-20-26/raw_I000_X1_C3.fits.SIM.fits", path "\\\\BIZ-SERVER\\Messdaten/Entwicklung/Tango/20180703_ISS-flug/AuswertungISS/010_2018-07-06_17-20-26/raw_I001_X0_C0.fits.SIM.fits", path "\\\\BIZ-SERVER\\Messdaten/Entwicklung/Tango/20180703_ISS-flug/AuswertungISS/010_2018-07-06_17-20-26/raw_I001_X0_C1.fits.SIM.fits", path "\\\\BIZ-SERVER\\Messdaten/Entwicklung/Tango/20180703_ISS-flug/AuswertungISS/010_2018-07-06_17-20-26/raw_I001_X0_C3.fits.SIM.fits", path "\\\\BIZ-SERVER\\Messdaten/Entwicklung/Tango/20180703_ISS-flug/AuswertungISS/011_2018-07-06_17-40-54/raw_I000_X0_C0.fits.SIM.fits", path "\\\\BIZ-SERVER\\Messdaten/Entwicklung/Tango/20180703_ISS-flug/AuswertungISS/011_2018-07-06_17-40-54/raw_I000_X0_C1.fits.SIM.fits", path "\\\\BIZ-SERVER\\Messdaten/Entwicklung/Tango/20180703_ISS-flug/AuswertungISS/011_2018-07-06_17-40-54/raw_I000_X0_C3.fits.SIM.fits", path "\\\\BIZ-SERVER\\Messdaten/Entwicklung/Tango/20180703_ISS-flug/AuswertungISS/011_2018-07-06_17-40-54/raw_I000_X1_C3.fits.SIM.fits", path "\\\\BIZ-SERVER\\Messdaten/Entwicklung/Tango/20180703_ISS-flug/AuswertungISS/011_2018-07-06_17-40-54/raw_I001_X1_C3.fits.SIM.fits", path "\\\\BIZ-SERVER\\Messdaten/Entwicklung/Tango/20180703_ISS-flug/AuswertungISS/011_2018-07-06_17-40-54/raw_I002_X1_C3.fits.SIM.fits", path "\\\\BIZ-SERVER\\Messdaten/Entwicklung/Tango/20180703_ISS-flug/AuswertungISS/011_2018-07-06_17-40-54/raw_I003_X1_C3.fits.SIM.fits", path "\\\\BIZ-SERVER\\Messdaten/Entwicklung/Tango/20180703_ISS-flug/AuswertungISS/011_2018-07-06_17-40-54/raw_I004_X1_C3.fits.SIM.fits", path "\\\\BIZ-SERVER\\Messdaten/Entwicklung/Tango/20180703_ISS-flug/AuswertungISS/011_2018-07-06_17-40-54/raw_I005_X1_C3.fits.SIM.fits", path "\\\\BIZ-SERVER\\Messdaten/Entwicklung/Tango/20180703_ISS-flug/AuswertungISS/011_2018-07-06_17-40-54/raw_I006_X1_C3.fits.SIM.fits", path "\\\\BIZ-SERVER\\Messdaten/Entwicklung/Tango/20180703_ISS-flug/AuswertungISS/011_2018-07-06_17-40-54/raw_I007_X1_C3.fits.SIM.fits", path "\\\\BIZ-SERVER\\Messdaten/Entwicklung/Tango/20180703_ISS-flug/AuswertungISS/011_2018-07-06_17-40-54/raw_I008_X1_C3.fits.SIM.fits", path "\\\\BIZ-SERVER\\Messdaten/Entwicklung/Tango/20180703_ISS-flug/AuswertungISS/012_2018-07-07_01-02-54/raw_I000_X0_C0.fits.SIM.fits", path "\\\\BIZ-SERVER\\Messdaten/Entwicklung/Tango/20180703_ISS-flug/AuswertungISS/012_2018-07-07_01-02-54/raw_I000_X0_C1.fits.SIM.fits", path "\\\\BIZ-SERVER\\Messdaten/Entwicklung/Tango/20180703_ISS-flug/AuswertungISS/012_2018-07-07_01-02-54/raw_I000_X0_C3.fits.SIM.fits", path "\\\\BIZ-SERVER\\Messdaten/Entwicklung/Tango/20180703_ISS-flug/AuswertungISS/012_2018-07-07_01-02-54/raw_I000_X1_C3.fits.SIM.fits", path "\\\\BIZ-SERVER\\Messdaten/Entwicklung/Tango/20180703_ISS-flug/AuswertungISS/012_2018-07-07_01-02-54/raw_I001_X1_C3.fits.SIM.fits", path "\\\\BIZ-SERVER\\Messdaten/Entwicklung/Tango/20180703_ISS-flug/AuswertungISS/012_2018-07-07_01-02-54/raw_I002_X1_C3.fits.SIM.fits", path "\\\\BIZ-SERVER\\Messdaten/Entwicklung/Tango/20180703_ISS-flug/AuswertungISS/012_2018-07-07_01-02-54/raw_I003_X1_C3.fits.SIM.fits", path "\\\\BIZ-SERVER\\Messdaten/Entwicklung/Tango/20180703_ISS-flug/AuswertungISS/012_2018-07-07_01-02-54/raw_I004_X1_C3.fits.SIM.fits", path "\\\\BIZ-SERVER\\Messdaten/Entwicklung/Tango/20180703_ISS-flug/AuswertungISS/012_2018-07-07_01-02-54/raw_I005_X1_C3.fits.SIM.fits", path "\\\\BIZ-SERVER\\Messdaten/Entwicklung/Tango/20180703_ISS-flug/AuswertungISS/012_2018-07-07_01-02-54/raw_I006_X1_C3.fits.SIM.fits", path "\\\\BIZ-SERVER\\Messdaten/Entwicklung/Tango/20180703_ISS-flug/AuswertungISS/013_2018-07-07_08-02-53/raw_I000_X0_C0.fits.SIM.fits", path "\\\\BIZ-SERVER\\Messdaten/Entwicklung/Tango/20180703_ISS-flug/AuswertungISS/013_2018-07-07_08-02-53/raw_I000_X0_C1.fits.SIM.fits", path "\\\\BIZ-SERVER\\Messdaten/Entwicklung/Tango/20180703_ISS-flug/AuswertungISS/013_2018-07-07_08-02-53/raw_I000_X0_C3.fits.SIM.fits", path "\\\\BIZ-SERVER\\Messdaten/Entwicklung/Tango/20180703_ISS-flug/AuswertungISS/013_2018-07-07_08-02-53/raw_I000_X1_C0.fits.SIM.fits", path "\\\\BIZ-SERVER\\Messdaten/Entwicklung/Tango/20180703_ISS-flug/AuswertungISS/013_2018-07-07_08-02-53/raw_I000_X1_C3.fits.SIM.fits", path "\\\\BIZ-SERVER\\Messdaten/Entwicklung/Tango/20180703_ISS-flug/AuswertungISS/013_2018-07-07_08-02-53/raw_I001_X1_C0.fits.SIM.fits", path "\\\\BIZ-SERVER\\Messdaten/Entwicklung/Tango/20180703_ISS-flug/AuswertungISS/013_2018-07-07_08-02-53/raw_I001_X1_C3.fits.SIM.fits", path "\\\\BIZ-SERVER\\Messdaten/Entwicklung/Tango/20180703_ISS-flug/AuswertungISS/013_2018-07-07_08-02-53/raw_I002_X1_C0.fits.SIM.fits", path "\\\\BIZ-SERVER\\Messdaten/Entwicklung/Tango/20180703_ISS-flug/AuswertungISS/013_2018-07-07_08-02-53/raw_I002_X1_C3.fits.SIM.fits", path "\\\\BIZ-SERVER\\Messdaten/Entwicklung/Tango/20180703_ISS-flug/AuswertungISS/013_2018-07-07_08-02-53/raw_I003_X1_C0.fits.SIM.fits", path "\\\\BIZ-SERVER\\Messdaten/Entwicklung/Tango/20180703_ISS-flug/AuswertungISS/013_2018-07-07_08-02-53/raw_I003_X1_C3.fits.SIM.fits", path "\\\\BIZ-SERVER\\Messdaten/Entwicklung/Tango/20180703_ISS-flug/AuswertungISS/013_2018-07-07_08-02-53/raw_I004_X1_C0.fits.SIM.fits", path "\\\\BIZ-SERVER\\Messdaten/Entwicklung/Tango/20180703_ISS-flug/AuswertungISS/013_2018-07-07_08-02-53/raw_I004_X1_C3.fits.SIM.fits", path "\\\\BIZ-SERVER\\Messdaten/Entwicklung/Tango/20180703_ISS-flug/AuswertungISS/013_2018-07-07_08-02-53/raw_I005_X1_C0.fits.SIM.fits", path "\\\\BIZ-SERVER\\Messdaten/Entwicklung/Tango/20180703_ISS-flug/AuswertungISS/013_2018-07-07_08-02-53/raw_I005_X1_C3.fits.SIM.fits", path "\\\\BIZ-SERVER\\Messdaten/Entwicklung/Tango/20180703_ISS-flug/AuswertungISS/013_2018-07-07_08-02-53/raw_I006_X1_C0.fits.SIM.fits", path "\\\\BIZ-SERVER\\Messdaten/Entwicklung/Tango/20180703_ISS-flug/AuswertungISS/013_2018-07-07_08-02-53/raw_I006_X1_C3.fits.SIM.fits", path "\\\\BIZ-SERVER\\Messdaten/Entwicklung/Tango/20180703_ISS-flug/AuswertungISS/013_2018-07-07_08-02-53/raw_I007_X1_C0.fits.SIM.fits", path "\\\\BIZ-SERVER\\Messdaten/Entwicklung/Tango/20180703_ISS-flug/AuswertungISS/013_2018-07-07_08-02-53/raw_I007_X1_C3.fits.SIM.fits", path "\\\\BIZ-SERVER\\Messdaten/Entwicklung/Tango/20180703_ISS-flug/AuswertungISS/013_2018-07-07_08-02-53/raw_I008_X1_C0.fits.SIM.fits", path "\\\\BIZ-SERVER\\Messdaten/Entwicklung/Tango/20180703_ISS-flug/AuswertungISS/013_2018-07-07_08-02-53/raw_I008_X1_C3.fits.SIM.fits", path "\\\\BIZ-SERVER\\Messdaten/Entwicklung/Tango/20180703_ISS-flug/AuswertungISS/013_2018-07-07_08-02-53/raw_I009_X1_C0.fits.SIM.fits", path "\\\\BIZ-SERVER\\Messdaten/Entwicklung/Tango/20180703_ISS-flug/AuswertungISS/013_2018-07-07_08-02-53/raw_I009_X1_C3.fits.SIM.fits", path "\\\\BIZ-SERVER\\Messdaten/Entwicklung/Tango/20180703_ISS-flug/AuswertungISS/013_2018-07-07_08-02-53/raw_I010_X1_C0.fits.SIM.fits", path "\\\\BIZ-SERVER\\Messdaten/Entwicklung/Tango/20180703_ISS-flug/AuswertungISS/013_2018-07-07_08-02-53/raw_I010_X1_C3.fits.SIM.fits", path "\\\\BIZ-SERVER\\Messdaten/Entwicklung/Tango/20180703_ISS-flug/AuswertungISS/013_2018-07-07_08-02-53/raw_I011_X1_C0.fits.SIM.fits", path "\\\\BIZ-SERVER\\Messdaten/Entwicklung/Tango/20180703_ISS-flug/AuswertungISS/013_2018-07-07_08-02-53/raw_I011_X1_C3.fits.SIM.fits", path "\\\\BIZ-SERVER\\Messdaten/Entwicklung/Tango/20180703_ISS-flug/AuswertungISS/013_2018-07-07_08-02-53/raw_I012_X1_C0.fits.SIM.fits", path "\\\\BIZ-SERVER\\Messdaten/Entwicklung/Tango/20180703_ISS-flug/AuswertungISS/013_2018-07-07_08-02-53/raw_I012_X1_C3.fits.SIM.fits", path "\\\\BIZ-SERVER\\Messdaten/Entwicklung/Tango/20180703_ISS-flug/AuswertungISS/013_2018-07-07_08-02-53/raw_I013_X1_C0.fits.SIM.fits", path "\\\\BIZ-SERVER\\Messdaten/Entwicklung/Tango/20180703_ISS-flug/AuswertungISS/013_2018-07-07_08-02-53/raw_I013_X1_C3.fits.SIM.fits", path "\\\\BIZ-SERVER\\Messdaten/Entwicklung/Tango/20180703_ISS-flug/AuswertungISS/013_2018-07-07_08-02-53/raw_I014_X1_C0.fits.SIM.fits", path "\\\\BIZ-SERVER\\Messdaten/Entwicklung/Tango/20180703_ISS-flug/AuswertungISS/013_2018-07-07_08-02-53/raw_I014_X1_C3.fits.SIM.fits", path "\\\\BIZ-SERVER\\Messdaten/Entwicklung/Tango/20180703_ISS-flug/AuswertungISS/013_2018-07-07_08-02-53/raw_I015_X1_C0.fits.SIM.fits", path "\\\\BIZ-SERVER\\Messdaten/Entwicklung/Tango/20180703_ISS-flug/AuswertungISS/013_2018-07-07_08-02-53/raw_I015_X1_C3.fits.SIM.fits", path "\\\\BIZ-SERVER\\Messdaten/Entwicklung/Tango/20180703_ISS-flug/AuswertungISS/013_2018-07-07_08-02-53/raw_I016_X1_C0.fits.SIM.fits", path "\\\\BIZ-SERVER\\Messdaten/Entwicklung/Tango/20180703_ISS-flug/AuswertungISS/013_2018-07-07_08-02-53/raw_I016_X1_C3.fits.SIM.fits", path "\\\\BIZ-SERVER\\Messdaten/Entwicklung/Tango/20180703_ISS-flug/AuswertungISS/013_2018-07-07_08-02-53/raw_I017_X1_C0.fits.SIM.fits", path "\\\\BIZ-SERVER\\Messdaten/Entwicklung/Tango/20180703_ISS-flug/AuswertungISS/013_2018-07-07_08-02-53/raw_I017_X1_C3.fits.SIM.fits", path "\\\\BIZ-SERVER\\Messdaten/Entwicklung/Tango/20180703_ISS-flug/AuswertungISS/013_2018-07-07_08-02-53/raw_I018_X1_C0.fits.SIM.fits", path "\\\\BIZ-SERVER\\Messdaten/Entwicklung/Tango/20180703_ISS-flug/AuswertungISS/013_2018-07-07_08-02-53/raw_I018_X1_C3.fits.SIM.fits", path "\\\\BIZ-SERVER\\Messdaten/Entwicklung/Tango/20180703_ISS-flug/AuswertungISS/013_2018-07-07_08-02-53/raw_I019_X1_C0.fits.SIM.fits", path "\\\\BIZ-SERVER\\Messdaten/Entwicklung/Tango/20180703_ISS-flug/AuswertungISS/013_2018-07-07_08-02-53/raw_I019_X1_C3.fits.SIM.fits", path "\\\\BIZ-SERVER\\Messdaten/Entwicklung/Tango/20180703_ISS-flug/AuswertungISS/013_2018-07-07_08-02-53/raw_I020_X1_C0.fits.SIM.fits", path "\\\\BIZ-SERVER\\Messdaten/Entwicklung/Tango/20180703_ISS-flug/AuswertungISS/013_2018-07-07_08-02-53/raw_I020_X1_C3.fits.SIM.fits", path "\\\\BIZ-SERVER\\Messdaten/Entwicklung/Tango/20180703_ISS-flug/AuswertungISS/013_2018-07-07_08-02-53/raw_I021_X1_C0.fits.SIM.fits", path "\\\\BIZ-SERVER\\Messdaten/Entwicklung/Tango/20180703_ISS-flug/AuswertungISS/013_2018-07-07_08-02-53/raw_I021_X1_C3.fits.SIM.fits", path "\\\\BIZ-SERVER\\Messdaten/Entwicklung/Tango/20180703_ISS-flug/AuswertungISS/013_2018-07-07_08-02-53/raw_I022_X1_C0.fits.SIM.fits", path "\\\\BIZ-SERVER\\Messdaten/Entwicklung/Tango/20180703_ISS-flug/AuswertungISS/013_2018-07-07_08-02-53/raw_I022_X1_C3.fits.SIM.fits", path "\\\\BIZ-SERVER\\Messdaten/Entwicklung/Tango/20180703_ISS-flug/AuswertungISS/013_2018-07-07_08-02-53/raw_I023_X1_C0.fits.SIM.fits", path "\\\\BIZ-SERVER\\Messdaten/Entwicklung/Tango/20180703_ISS-flug/AuswertungISS/013_2018-07-07_08-02-53/raw_I023_X1_C3.fits.SIM.fits", path "\\\\BIZ-SERVER\\Messdaten/Entwicklung/Tango/20180703_ISS-flug/AuswertungISS/013_2018-07-07_08-02-53/raw_I024_X1_C0.fits.SIM.fits", path "\\\\BIZ-SERVER\\Messdaten/Entwicklung/Tango/20180703_ISS-flug/AuswertungISS/013_2018-07-07_08-02-53/raw_I024_X1_C3.fits.SIM.fits", path "\\\\BIZ-SERVER\\Messdaten/Entwicklung/Tango/20180703_ISS-flug/AuswertungISS/013_2018-07-07_08-02-53/raw_I025_X1_C0.fits.SIM.fits", path "\\\\BIZ-SERVER\\Messdaten/Entwicklung/Tango/20180703_ISS-flug/AuswertungISS/013_2018-07-07_08-02-53/raw_I025_X1_C3.fits.SIM.fits", path "\\\\BIZ-SERVER\\Messdaten/Entwicklung/Tango/20180703_ISS-flug/AuswertungISS/013_2018-07-07_08-02-53/raw_I026_X1_C0.fits.SIM.fits", path "\\\\BIZ-SERVER\\Messdaten/Entwicklung/Tango/20180703_ISS-flug/AuswertungISS/013_2018-07-07_08-02-53/raw_I026_X1_C3.fits.SIM.fits", path "\\\\BIZ-SERVER\\Messdaten/Entwicklung/Tango/20180703_ISS-flug/AuswertungISS/013_2018-07-07_08-02-53/raw_I027_X1_C0.fits.SIM.fits", path "\\\\BIZ-SERVER\\Messdaten/Entwicklung/Tango/20180703_ISS-flug/AuswertungISS/013_2018-07-07_08-02-53/raw_I027_X1_C3.fits.SIM.fits", path "\\\\BIZ-SERVER\\Messdaten/Entwicklung/Tango/20180703_ISS-flug/AuswertungISS/013_2018-07-07_08-02-53/raw_I028_X1_C0.fits.SIM.fits", path "\\\\BIZ-SERVER\\Messdaten/Entwicklung/Tango/20180703_ISS-flug/AuswertungISS/013_2018-07-07_08-02-53/raw_I028_X1_C3.fits.SIM.fits", path "\\\\BIZ-SERVER\\Messdaten/Entwicklung/Tango/20180703_ISS-flug/AuswertungISS/013_2018-07-07_08-02-53/raw_I029_X1_C0.fits.SIM.fits", path "\\\\BIZ-SERVER\\Messdaten/Entwicklung/Tango/20180703_ISS-flug/AuswertungISS/013_2018-07-07_08-02-53/raw_I029_X1_C3.fits.SIM.fits", path "\\\\BIZ-SERVER\\Messdaten/Entwicklung/Tango/20180703_ISS-flug/AuswertungISS/014_2018-07-16_17-53-52/raw_I000_X0_C0.fits.SIM.fits", path "\\\\BIZ-SERVER\\Messdaten/Entwicklung/Tango/20180703_ISS-flug/AuswertungISS/014_2018-07-16_17-53-52/raw_I000_X0_C1.fits.SIM.fits", path "\\\\BIZ-SERVER\\Messdaten/Entwicklung/Tango/20180703_ISS-flug/AuswertungISS/014_2018-07-16_17-53-52/raw_I000_X0_C3.fits.SIM.fits", path "\\\\BIZ-SERVER\\Messdaten/Entwicklung/Tango/20180703_ISS-flug/AuswertungISS/014_2018-07-16_17-53-52/raw_I000_X1_C0.fits.SIM.fits", path "\\\\BIZ-SERVER\\Messdaten/Entwicklung/Tango/20180703_ISS-flug/AuswertungISS/014_2018-07-16_17-53-52/raw_I000_X1_C3.fits.SIM.fits", path "\\\\BIZ-SERVER\\Messdaten/Entwicklung/Tango/20180703_ISS-flug/AuswertungISS/014_2018-07-16_17-53-52/raw_I001_X1_C0.fits.SIM.fits", path "\\\\BIZ-SERVER\\Messdaten/Entwicklung/Tango/20180703_ISS-flug/AuswertungISS/014_2018-07-16_17-53-52/raw_I001_X1_C3.fits.SIM.fits", path "\\\\BIZ-SERVER\\Messdaten/Entwicklung/Tango/20180703_ISS-flug/AuswertungISS/014_2018-07-16_17-53-52/raw_I002_X1_C0.fits.SIM.fits", path "\\\\BIZ-SERVER\\Messdaten/Entwicklung/Tango/20180703_ISS-flug/AuswertungISS/014_2018-07-16_17-53-52/raw_I002_X1_C3.fits.SIM.fits", path "\\\\BIZ-SERVER\\Messdaten/Entwicklung/Tango/20180703_ISS-flug/AuswertungISS/014_2018-07-16_17-53-52/raw_I003_X1_C0.fits.SIM.fits", path "\\\\BIZ-SERVER\\Messdaten/Entwicklung/Tango/20180703_ISS-flug/AuswertungISS/014_2018-07-16_17-53-52/raw_I003_X1_C3.fits.SIM.fits", path "\\\\BIZ-SERVER\\Messdaten/Entwicklung/Tango/20180703_ISS-flug/AuswertungISS/014_2018-07-16_17-53-52/raw_I004_X1_C0.fits.SIM.fits", path "\\\\BIZ-SERVER\\Messdaten/Entwicklung/Tango/20180703_ISS-flug/AuswertungISS/014_2018-07-16_17-53-52/raw_I004_X1_C3.fits.SIM.fits", path "\\\\BIZ-SERVER\\Messdaten/Entwicklung/Tango/20180703_ISS-flug/AuswertungISS/014_2018-07-16_17-53-52/raw_I005_X1_C0.fits.SIM.fits", path "\\\\BIZ-SERVER\\Messdaten/Entwicklung/Tango/20180703_ISS-flug/AuswertungISS/014_2018-07-16_17-53-52/raw_I005_X1_C3.fits.SIM.fits", path "\\\\BIZ-SERVER\\Messdaten/Entwicklung/Tango/20180703_ISS-flug/AuswertungISS/014_2018-07-16_17-53-52/raw_I006_X1_C0.fits.SIM.fits", path "\\\\BIZ-SERVER\\Messdaten/Entwicklung/Tango/20180703_ISS-flug/AuswertungISS/014_2018-07-16_17-53-52/raw_I006_X1_C3.fits.SIM.fits", path "\\\\BIZ-SERVER\\Messdaten/Entwicklung/Tango/20180703_ISS-flug/AuswertungISS/014_2018-07-16_17-53-52/raw_I007_X1_C0.fits.SIM.fits", path "\\\\BIZ-SERVER\\Messdaten/Entwicklung/Tango/20180703_ISS-flug/AuswertungISS/014_2018-07-16_17-53-52/raw_I007_X1_C3.fits.SIM.fits", path "\\\\BIZ-SERVER\\Messdaten/Entwicklung/Tango/20180703_ISS-flug/AuswertungISS/014_2018-07-16_17-53-52/raw_I008_X1_C0.fits.SIM.fits", path "\\\\BIZ-SERVER\\Messdaten/Entwicklung/Tango/20180703_ISS-flug/AuswertungISS/014_2018-07-16_17-53-52/raw_I008_X1_C3.fits.SIM.fits", path "\\\\BIZ-SERVER\\Messdaten/Entwicklung/Tango/20180703_ISS-flug/AuswertungISS/014_2018-07-16_17-53-52/raw_I009_X1_C0.fits.SIM.fits", path "\\\\BIZ-SERVER\\Messdaten/Entwicklung/Tango/20180703_ISS-flug/AuswertungISS/014_2018-07-16_17-53-52/raw_I009_X1_C3.fits.SIM.fits", path "\\\\BIZ-SERVER\\Messdaten/Entwicklung/Tango/20180703_ISS-flug/AuswertungISS/014_2018-07-16_17-53-52/raw_I010_X1_C0.fits.SIM.fits", path "\\\\BIZ-SERVER\\Messdaten/Entwicklung/Tango/20180703_ISS-flug/AuswertungISS/014_2018-07-16_17-53-52/raw_I010_X1_C3.fits.SIM.fits", path "\\\\BIZ-SERVER\\Messdaten/Entwicklung/Tango/20180703_ISS-flug/AuswertungISS/014_2018-07-16_17-53-52/raw_I011_X1_C0.fits.SIM.fits", path "\\\\BIZ-SERVER\\Messdaten/Entwicklung/Tango/20180703_ISS-flug/AuswertungISS/014_2018-07-16_17-53-52/raw_I011_X1_C3.fits.SIM.fits", path "\\\\BIZ-SERVER\\Messdaten/Entwicklung/Tango/20180703_ISS-flug/AuswertungISS/014_2018-07-16_17-53-52/raw_I012_X1_C0.fits.SIM.fits", path "\\\\BIZ-SERVER\\Messdaten/Entwicklung/Tango/20180703_ISS-flug/AuswertungISS/014_2018-07-16_17-53-52/raw_I012_X1_C3.fits.SIM.fits", path "\\\\BIZ-SERVER\\Messdaten/Entwicklung/Tango/20180703_ISS-flug/AuswertungISS/014_2018-07-16_17-53-52/raw_I013_X1_C0.fits.SIM.fits", path "\\\\BIZ-SERVER\\Messdaten/Entwicklung/Tango/20180703_ISS-flug/AuswertungISS/014_2018-07-16_17-53-52/raw_I013_X1_C3.fits.SIM.fits", path "\\\\BIZ-SERVER\\Messdaten/Entwicklung/Tango/20180703_ISS-flug/AuswertungISS/014_2018-07-16_17-53-52/raw_I014_X1_C0.fits.SIM.fits", path "\\\\BIZ-SERVER\\Messdaten/Entwicklung/Tango/20180703_ISS-flug/AuswertungISS/014_2018-07-16_17-53-52/raw_I014_X1_C3.fits.SIM.fits", path "\\\\BIZ-SERVER\\Messdaten/Entwicklung/Tango/20180703_ISS-flug/AuswertungISS/014_2018-07-16_17-53-52/raw_I015_X1_C0.fits.SIM.fits", path "\\\\BIZ-SERVER\\Messdaten/Entwicklung/Tango/20180703_ISS-flug/AuswertungISS/014_2018-07-16_17-53-52/raw_I015_X1_C3.fits.SIM.fits", path "\\\\BIZ-SERVER\\Messdaten/Entwicklung/Tango/20180703_ISS-flug/AuswertungISS/014_2018-07-16_17-53-52/raw_I016_X1_C0.fits.SIM.fits", path "\\\\BIZ-SERVER\\Messdaten/Entwicklung/Tango/20180703_ISS-flug/AuswertungISS/014_2018-07-16_17-53-52/raw_I016_X1_C3.fits.SIM.fits", path "\\\\BIZ-SERVER\\Messdaten/Entwicklung/Tango/20180703_ISS-flug/AuswertungISS/014_2018-07-16_17-53-52/raw_I017_X1_C0.fits.SIM.fits", path "\\\\BIZ-SERVER\\Messdaten/Entwicklung/Tango/20180703_ISS-flug/AuswertungISS/014_2018-07-16_17-53-52/raw_I017_X1_C3.fits.SIM.fits", path "\\\\BIZ-SERVER\\Messdaten/Entwicklung/Tango/20180703_ISS-flug/AuswertungISS/014_2018-07-16_17-53-52/raw_I018_X1_C0.fits.SIM.fits", path "\\\\BIZ-SERVER\\Messdaten/Entwicklung/Tango/20180703_ISS-flug/AuswertungISS/014_2018-07-16_17-53-52/raw_I018_X1_C3.fits.SIM.fits", path "\\\\BIZ-SERVER\\Messdaten/Entwicklung/Tango/20180703_ISS-flug/AuswertungISS/014_2018-07-16_17-53-52/raw_I019_X1_C0.fits.SIM.fits", path "\\\\BIZ-SERVER\\Messdaten/Entwicklung/Tango/20180703_ISS-flug/AuswertungISS/014_2018-07-16_17-53-52/raw_I019_X1_C3.fits.SIM.fits", path "\\\\BIZ-SERVER\\Messdaten/Entwicklung/Tango/20180703_ISS-flug/AuswertungISS/014_2018-07-16_17-53-52/raw_I020_X1_C0.fits.SIM.fits", path "\\\\BIZ-SERVER\\Messdaten/Entwicklung/Tango/20180703_ISS-flug/AuswertungISS/014_2018-07-16_17-53-52/raw_I020_X1_C3.fits.SIM.fits", path "\\\\BIZ-SERVER\\Messdaten/Entwicklung/Tango/20180703_ISS-flug/AuswertungISS/014_2018-07-16_17-53-52/raw_I021_X1_C0.fits.SIM.fits", path "\\\\BIZ-SERVER\\Messdaten/Entwicklung/Tango/20180703_ISS-flug/AuswertungISS/014_2018-07-16_17-53-52/raw_I021_X1_C3.fits.SIM.fits", path "\\\\BIZ-SERVER\\Messdaten/Entwicklung/Tango/20180703_ISS-flug/AuswertungISS/014_2018-07-16_17-53-52/raw_I022_X1_C0.fits.SIM.fits", path "\\\\BIZ-SERVER\\Messdaten/Entwicklung/Tango/20180703_ISS-flug/AuswertungISS/014_2018-07-16_17-53-52/raw_I022_X1_C3.fits.SIM.fits", path "\\\\BIZ-SERVER\\Messdaten/Entwicklung/Tango/20180703_ISS-flug/AuswertungISS/014_2018-07-16_17-53-52/raw_I023_X1_C0.fits.SIM.fits", path "\\\\BIZ-SERVER\\Messdaten/Entwicklung/Tango/20180703_ISS-flug/AuswertungISS/014_2018-07-16_17-53-52/raw_I023_X1_C3.fits.SIM.fits", path "\\\\BIZ-SERVER\\Messdaten/Entwicklung/Tango/20180703_ISS-flug/AuswertungISS/014_2018-07-16_17-53-52/raw_I024_X1_C0.fits.SIM.fits", path "\\\\BIZ-SERVER\\Messdaten/Entwicklung/Tango/20180703_ISS-flug/AuswertungISS/014_2018-07-16_17-53-52/raw_I024_X1_C3.fits.SIM.fits", path "\\\\BIZ-SERVER\\Messdaten/Entwicklung/Tango/20180703_ISS-flug/AuswertungISS/014_2018-07-16_17-53-52/raw_I025_X1_C0.fits.SIM.fits", path "\\\\BIZ-SERVER\\Messdaten/Entwicklung/Tango/20180703_ISS-flug/AuswertungISS/014_2018-07-16_17-53-52/raw_I025_X1_C3.fits.SIM.fits", path "\\\\BIZ-SERVER\\Messdaten/Entwicklung/Tango/20180703_ISS-flug/AuswertungISS/014_2018-07-16_17-53-52/raw_I026_X1_C0.fits.SIM.fits", path "\\\\BIZ-SERVER\\Messdaten/Entwicklung/Tango/20180703_ISS-flug/AuswertungISS/014_2018-07-16_17-53-52/raw_I026_X1_C3.fits.SIM.fits", path "\\\\BIZ-SERVER\\Messdaten/Entwicklung/Tango/20180703_ISS-flug/AuswertungISS/014_2018-07-16_17-53-52/raw_I027_X1_C0.fits.SIM.fits", path "\\\\BIZ-SERVER\\Messdaten/Entwicklung/Tango/20180703_ISS-flug/AuswertungISS/014_2018-07-16_17-53-52/raw_I027_X1_C3.fits.SIM.fits", path "\\\\BIZ-SERVER\\Messdaten/Entwicklung/Tango/20180703_ISS-flug/AuswertungISS/014_2018-07-16_17-53-52/raw_I028_X1_C0.fits.SIM.fits", path "\\\\BIZ-SERVER\\Messdaten/Entwicklung/Tango/20180703_ISS-flug/AuswertungISS/014_2018-07-16_17-53-52/raw_I028_X1_C3.fits.SIM.fits", path "\\\\BIZ-SERVER\\Messdaten/Entwicklung/Tango/20180703_ISS-flug/AuswertungISS/014_2018-07-16_17-53-52/raw_I029_X1_C0.fits.SIM.fits", path "\\\\BIZ-SERVER\\Messdaten/Entwicklung/Tango/20180703_ISS-flug/AuswertungISS/014_2018-07-16_17-53-52/raw_I029_X1_C3.fits.SIM.fits"]
  # "this is maximum in X-direction!"
  # "use Recusrive File List"
  # "epi ~65000/8000= 8\nSIM ~65000/2000=32"
  # "Pfad muss existieren sonst fehler 1"
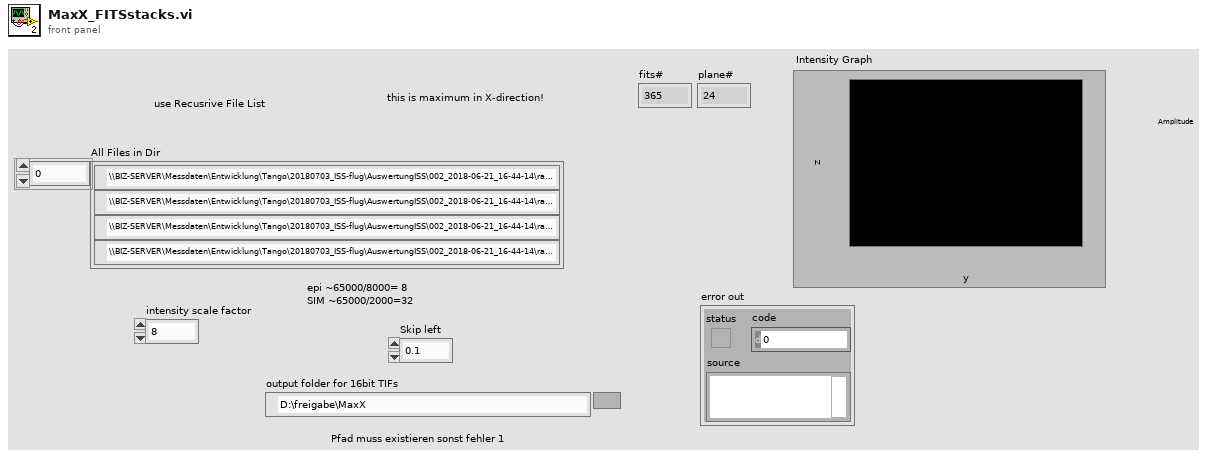
[diagram p1: front panel]
types:
  T1 = cluster{"fits refnum":refnum<file>, "Byte-Reihenfolge (0:Big-Endian, 2:LSB)":enum16{"big-endian, network order", "native, host order", "little-endian"}}
  T2 = cluster{"BITPIX":i16, "NAXIS":i16, "NAXIS1":u16, "NAXIS2":u16, "NAXIS3":u16, "BZERO":dbl, "BSCALE":dbl}
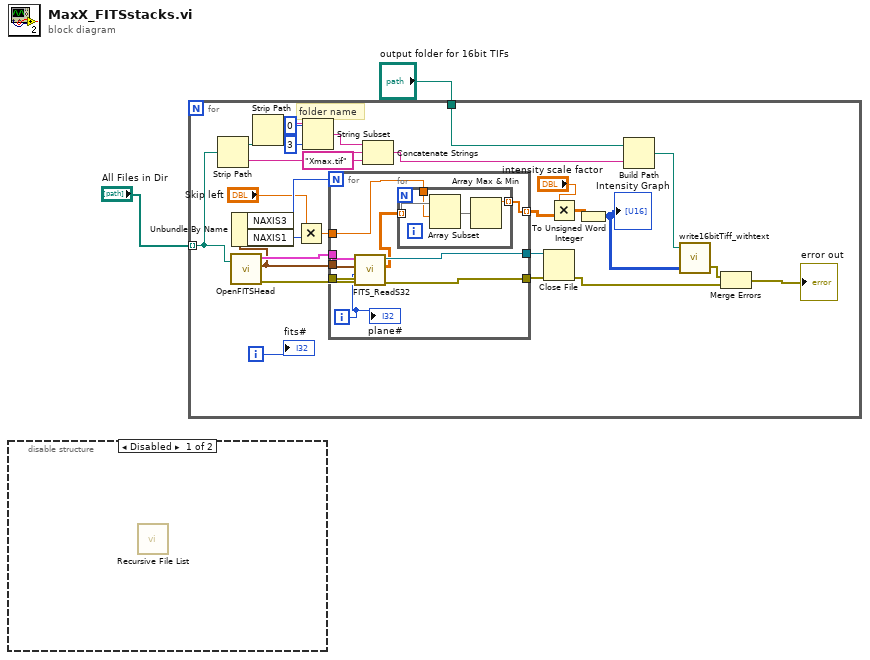
[diagram p0: block diagram]
diagram:
  n1 = disable-structure shown="Disabled" {
    frame Disabled {
      n2 = call <vilib>:"Recursive File List.vi"() -> ()  [unwired: 7 in, 5 out]
    }
    frame Enabled {
    }
  }
  n3 = for {
    tunnel: "All Files in Dir" -> [w24] mode=indexing
    tunnel: "output folder for 16bit TIFs" -> [w20]
    i -> [w30]
    # "folder name"
    n4 = Strip Path(path=w24) -> (stripped path=w12:path, name=w23:string)
    n5 = call "OpenFITSHead.vi"("file path"=w24) -> ("FITS file"=w26:T1, "FITS"=w25:T2, "error out"=w6:errorcluster)  [unwired: 2 in]
    n6 = Unbundle By Name(w25) -> ("NAXIS3"=w7:u16, "NAXIS1"=w5:u16)
    n7 = Strip Path(path=w12) -> (name=w11:string)  [unwired: 1 out]
    n8 = Multiply(x="Skip left", y=w5) -> (x*y=w3:dbl)
    n9 = String Subset(string=w11, offset (0)=0, length (rest)=3 ("length (rest)")) -> (substring=w8:string)
    n10 = for {
      N: w7 -> [_]
      tunnel: w26 -> [w39]
      tunnel: w6 -> [w38]
      tunnel: w25 -> [w37]
      tunnel: [w36] -> w29
      tunnel: [w35] -> w28
      tunnel: [w32] -> w27 mode=indexing
      tunnel: w3 -> [w31]
      i -> [w34]
      n11 = call "FITS_ReadS32.vi"("error in (no error)"=w38, "Plane# (0..n-1)"=w34, "FITS"=w37, "FITS file"=w39) -> ("error out"=w35:errorcluster, "Array"=w33:sgl[][], "Byte Stream File out"=w36:refnum<file>)  [unwired: 5 in]
      n12 = for {
        tunnel: w33 -> [w42] mode=indexing
        tunnel: [w43] -> w32 mode=indexing
        tunnel: w31 -> [w40]
        n13 = Array Subset(array=w42, index=w40) -> (w41:sgl[])  [unwired: 1 in]
        n14 = Array Max & Min(array=w41) -> (max value=w43:sgl)  [unwired: 3 out]
      }
      "plane#" <- w34
    }
    n15 = Concatenate Strings(w8, w23, "Xmax.tif" ("string")) -> (w21:string)
    n16 = Close File(refnum=w29, error in=w28) -> (error out=w14:errorcluster)  [unwired: 1 out]
    n17 = Multiply(x="intensity scale factor", y=w27) -> (x*y=w19:dbl[][])
    n18 = To Unsigned Word Integer(number=w19) -> (unsigned 16bit integer=w17:u16[][])
    "Intensity Graph" <- w17
    n19 = Build Path(base path=w20, name or relative path=w21) -> (appended path=w16:path)
    n20 = call "write16bitTiff_withtext.vi"("16-bit pixmap x, y"=w17, "file path"=w16) -> ("error out"=w15:errorcluster)  [unwired: 2 in]
    n21 = Merge Errors(w15, w14) -> (→"error out":errorcluster)
    "fits#" <- w30
  }
